vi "CloseBling.vi"(5 "Turn off LEDs on close":bool=TRUE, 8 "error in (no error)":errorcluster, 11 "ControlState in":T1 {"ChainMask" format="0x%02x"}) -> (0 "error out":errorcluster)   [LabVIEW 2018, in "ArduinoSerialBling.lvlib"]
uses:
  ArduinoSerialBling.lvlib
  ControlState.ctl
  ConnectionType.ctl
  UdpConnection.ctl
  ChainState.ctl
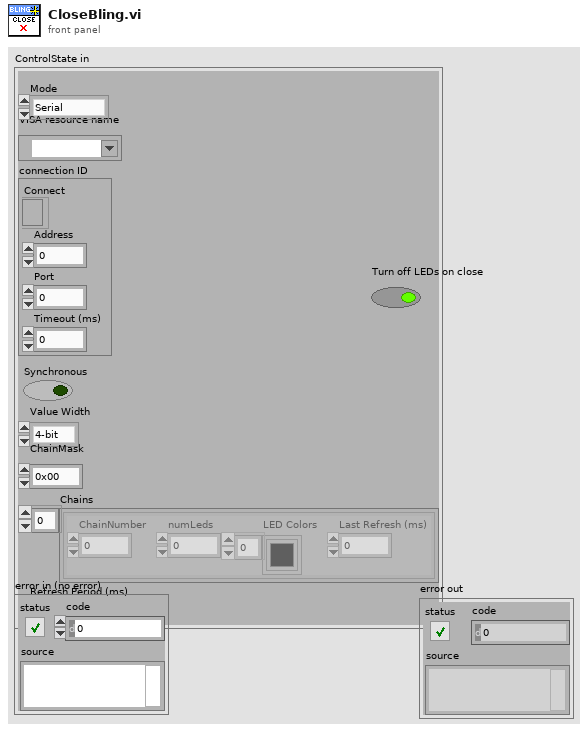
[diagram p1: front panel]
types:
  T1 = typedef "ArduinoSerialBling.lvlib/ControlState.ctl" = cluster{"Mode":T2, "VISA resource name":refnum<visa-resource-name>, "connection ID":T3, "Synchronous":bool, "Value Width":enum16{"4-bit", "8-bit"}, "ChainMask":u8, "Chains":T4[], "Refresh Period (ms)":u32}
  T2 = typedef "ConnectionType.ctl" = enum16{"Serial", "Ethernet", "Offline"}
  T3 = typedef "UdpConnection.ctl" = cluster{"Connect":refnum<k16>, "Address":u32, "Port":u16, "Timeout (ms)":i32}
  T4 = typedef "ArduinoSerialBling.lvlib/ChainState.ctl" = cluster{"ChainNumber":u8, "numLeds":u8, "LED Colors":u32[], "Last Refresh (ms)":u32}
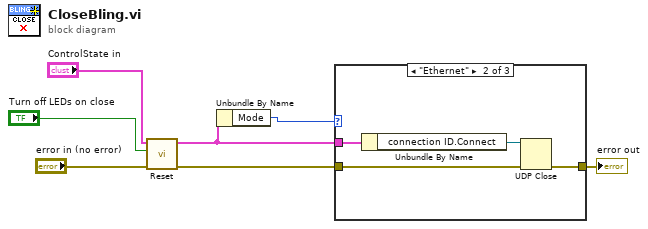
[diagram p0: block diagram]
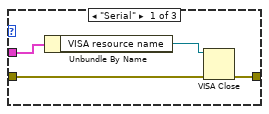
[diagram p2: hidden frame]
diagram:
  n1 = call "Reset.vi"("error in (no error)"="error in (no error)", "Reset"="Turn off LEDs on close", "ControlState in"="ControlState in") -> ("error out"=w4:errorcluster, "ControlState out"=w2:T1)  [unwired: 7 in]
  n2 = Unbundle By Name(w2) -> ("Mode"=w1:T2)
  n3 = case shown="\"Ethernet\"" w1 {
    tunnel: [w10 w15 w16] -> w7
    tunnel: w2 -> [w9 w14 _]
    tunnel: w4 -> [w8 w12 w16]
    frame "Serial" {
      n4 = Unbundle By Name(w9) -> ("VISA resource name"=w11:refnum<visa-resource-name>)
      n5 = VISA Close(VISA resource name=w11, error in (no error)=w8) -> (error out=w10:errorcluster)
    }
    frame "Ethernet" {
      n6 = Unbundle By Name(w14) -> ("connection ID.Connect"=w13:refnum<k16>)
      n7 = UDP Close(connection ID=w13, 8:w12) -> (error out=w15:errorcluster)  [unwired: 1 out]
    }
    frame "Offline", Default {
    }
  }
  "error out" <- w7
